vi "FGC.vi"(0 "System no.":i32=1 min=1 max=4 step=1, 1 "Routine name":string, 2 "Scan axis value":dbl format="%.6f", 3 "Step axis value":dbl format="%.6f", 4 "No.of digits":i16=6, 5 "error in":errorcluster, 7 "Single axis scan?":bool) -> (19 "error out":errorcluster)   [LabVIEW 2020]
doc: "Sets fast alignment gradient search dither center: \nIf only one axis is used for the routine, \"Step Axis Value\" will be set identical to \"Scan Axis Value\".\n\nC-887, E-712:"
panel:
  # "Sets Fast Gradient scan dither Center"
  # "FGC parameters"
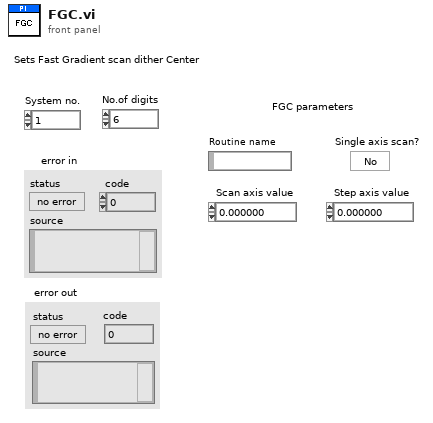
[diagram p1: front panel]
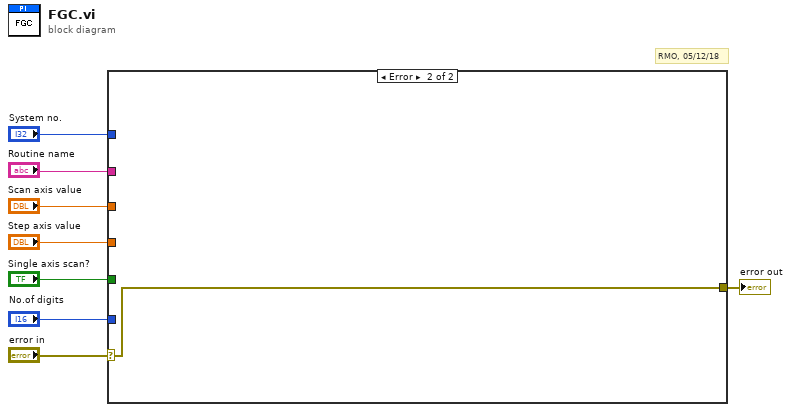
[diagram p0: block diagram]
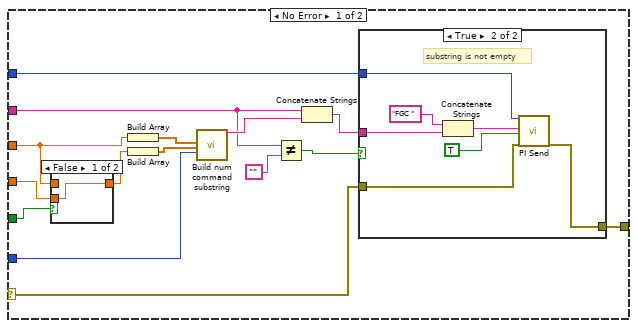
[diagram p2: hidden frame]
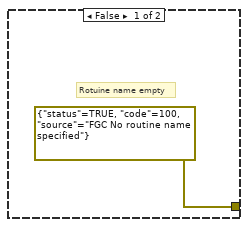
[diagram p4: hidden frame]
diagram:
  # "RMO, 05/12/18"
  n1 = case shown="Error" "error in" {
    selector: "error in" -> [w9 w34]
    tunnel: [w23 w34] -> w8
    tunnel: "No.of digits" -> [w21 _]
    tunnel: "System no." -> [w22 _]
    tunnel: "Routine name" -> [w16 _]
    tunnel: "Scan axis value" -> [w12 _]
    tunnel: "Step axis value" -> [w13 _]
    tunnel: "Single axis scan?" -> [w14 _]
    frame No Error {
      n2 = case shown="False" w14 {
        tunnel: w13 -> [w24 _]
        tunnel: w12 -> [_ w25]
        tunnel: [w24 w25] -> w11
        frame False {
        }
        frame True {
        }
      }
      n3 = Build Array(w12) -> (w20:dbl[])
      n4 = Build Array(w11) -> (w19:dbl[])
      n5 = call "Build num command substring.vi"("Num 1"=w20, "Num 2"=w19, "No. of digits"=w21) -> ("Command substring"=w18:string)  [unwired: 16 out]
      n6 = Not Equal?(x=w16, y="") -> (x != y?=w10:bool)
      n7 = Concatenate Strings(w16, w18) -> (w17:string)
      n8 = case shown="True" w10 {
        tunnel: [errorcluster {"status"=TRUE, "code"=100, "source"="FGC No routine name specified"} ("error out") w30] -> w23
        tunnel: w22 -> [_ w29]
        tunnel: w17 -> [_ w28]
        tunnel: w9 -> [_ w27]
        frame False {
          # "Rotuine name empty"
        }
        frame True {
          # "substring is not empty"
          n9 = Concatenate Strings("FGC ", w28) -> (w31:string)
          n10 = call "PI Send.vi"("System no."=w29, "String to send"=w31, "Attach termination char.?"=TRUE ("Attach Linefeed?"), "error in"=w27) -> ("error out"=w30:errorcluster)  [unwired: 2 in, 13 out]
        }
      }
    }
    frame Error {
    }
  }
  "error out" <- w8
